vi "Flow vs Int Fac Input.vi"() -> ()   [LabVIEW 2009]
uses:
  Intellifaucet/Intellfaucet Mode.ctl
  ChannelSettings.ctl
  <vilib>/Analysis/NI_AALBase.lvlib
panel:
  out "Results(Flow,Percent)":dbl[][](array[numeric])
  out "Flowrate":dbl(graph)
  out "Percent Input":i32
  out "error out":errorcluster
  out "Flow":dbl
  in  "seconds to wait between reported averages":u32=15
  in  "error in (no error)":errorcluster
  in  "Semiphore":T1
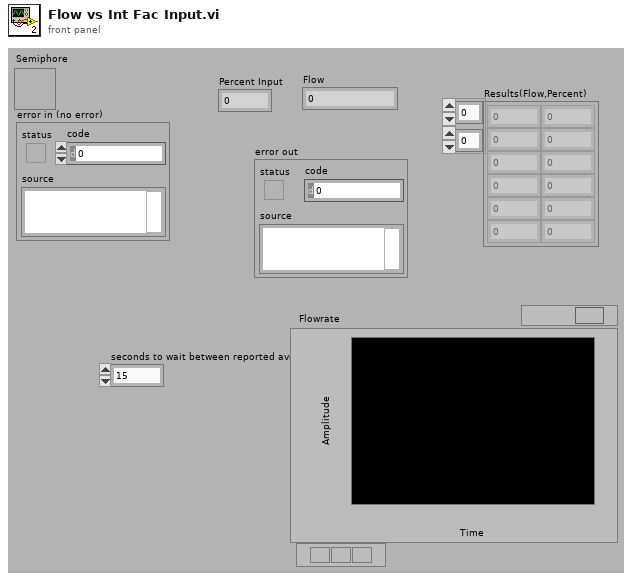
[diagram p1: front panel]
types:
  T1 = typedef "Semaphore RefNum" = refnum<k1>
  T2 = typedef "Intellfaucet Mode.ctl" = enum16{"Adjust Temp", "Adjust Flow", "Start Flow", "Stop Flow"}
  T3 = typedef "ChannelSettings.ctl" = u32
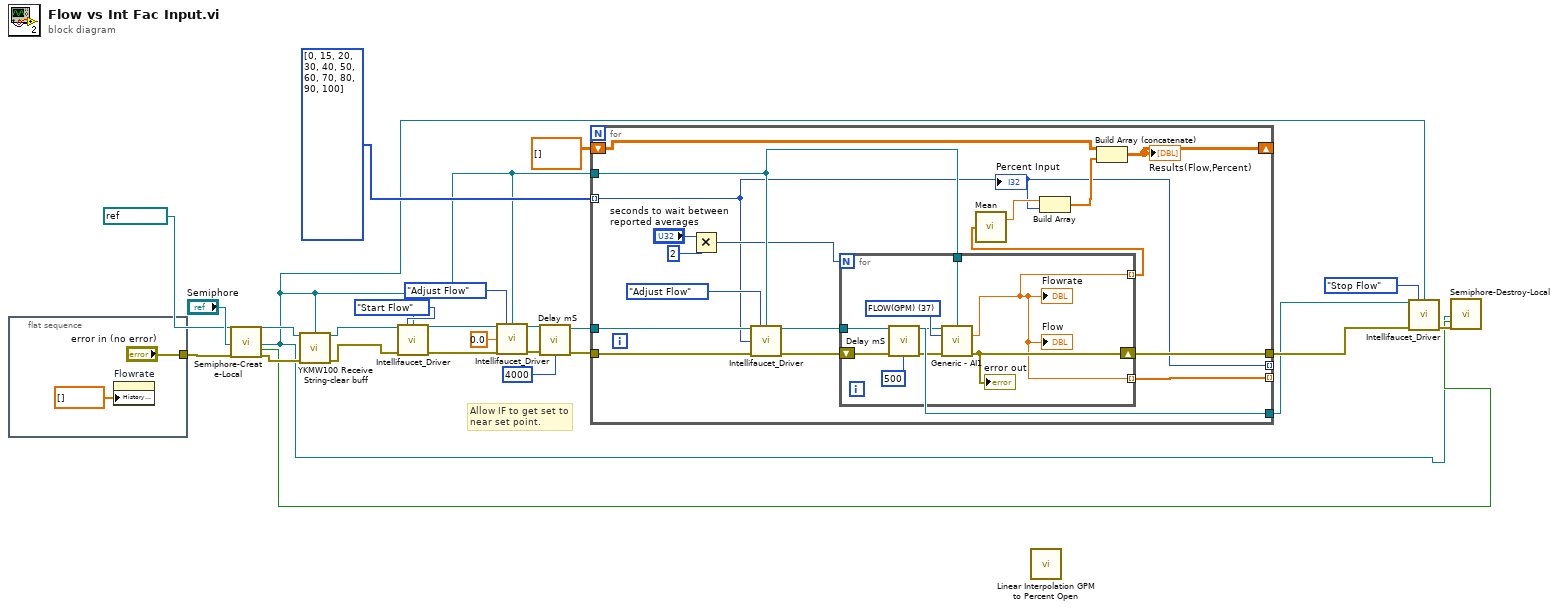
[diagram p0: block diagram]
diagram:
  # "Allow IF to get set to\nnear set point."
  n1 = flat-sequence {
    tunnel: ["error in (no error)"] -> w22
    frame #0 {
      n2 = property on="Flowrate" class="WFChart (strict)"("History Data"=dbl[] []) -> ()  [unwired: 2 in, 2 out]
    }
  }
  n3 = call "Semiphore-Create-Local.vi"("Semiphore"="Semiphore", "error in (no error)"=w22) -> ("semaphore"=w4:T1, "Local?"=w13:bool, "error out"=w15:errorcluster)  [unwired: 15 in]
  n4 = call "YKMW100 Receive String-clear buff.vi"("VISA session"=refnum<visa-resource-name> "MW100" ("MW100"), "Semiphore"=w4, "error in (no error)"=w15) -> ("dup VISA session"=w11:refnum<visa-resource-name>, "error out"=w14:errorcluster)  [unwired: 10 in, 1 out]
  n5 = call "Intellifaucet_Driver.vi"("VISA session"=w11, "Mode"=Intellfaucet_Mode."Start Flow", "Semiphore"=w4, "Error In"=w14) -> ("VISA session out"=w5:refnum<visa-resource-name>, "Error Out"=w10:errorcluster)  [unwired: 10 in]
  n6 = call "Intellifaucet_Driver.vi"("VISA session"=w5, "Mode"=Intellfaucet_Mode."Adjust Flow", "Semiphore"=w4, "Percent Flow"=0.0, "Error In"=w10) -> ("VISA session out"=w7:refnum<visa-resource-name>, "Error Out"=w9:errorcluster)  [unwired: 9 in]
  n7 = call "Delay mS.vi"("Error In"=w9, "milliseconds to wait"=u32 4000) -> ("Error Out"=w8:errorcluster)  [unwired: 13 in]
  n8 = for {
    tunnel: [w37] -> _ mode=indexing
    tunnel: w8 -> [w40]
    tunnel: w4 -> [w39]
    tunnel: [w28] -> _ mode=indexing
    tunnel: [w42] -> w18
    tunnel: i32[] [0, 15, 20, 30, 40, 50, 60, 70, 80, 90, 100] -> [w28] mode=indexing
    tunnel: [w36] -> w17
    tunnel: w7 -> [w35]
    shift-right: [w27] -> _
    shift-left: dbl[][] [] -> [w26]
    n9 = Multiply(x="seconds to wait between reported averages", y=u32 2) -> (x*y=w32:u32)
    n10 = call "Intellifaucet_Driver.vi"("VISA session"=w35, "Mode"=Intellfaucet_Mode."Adjust Flow", "Semiphore"=w39, "Percent Flow"=w28, "Error In"=w40) -> ("VISA session out"=w36:refnum<visa-resource-name>, "Error Out"=w41:errorcluster)  [unwired: 9 in]
    n11 = for {
      N: w32 -> [_]
      tunnel: w39 -> [w46]
      tunnel: [w43] -> w37 mode=indexing
      tunnel: w36 -> [w45]
      shift-right: [w48] -> w42
      shift-left: w41 -> [w47]
      tunnel: [w43] -> w31 mode=indexing
      w50 = T3 37 items=["4-20_OUT", "Pres_HI1", "Pres_HI2", "Pres_LOW", "Pres_PIN", "HEATER_TOP", "HEATER_BOT", "T_Shell", "FLOWMETER", "WATT_SENSE", "WH_TICK", "Tc_1", "Tc_2", "Tc_3", "Tc_4", "Tc_5", "Tc_6", "Tc_down", "T_Shell_2", "T_Shell_3", "T_Shell_4", "RTD_IN", "RTD_OUT", "RTD_AMB", "INTF_TEMPFLO", "INTF_READY", "INTF_START", "INTF_STOP", "DRM_LOW", "DRM_HIGH", "PWR_MAIN", "VLV_DUMP", "VLV_OUT", "VLV_IN", "WATT_HOURS", "FLOW(SAMPLE)", "GALLONS", "FLOW(GPM)"] ("Channel_Enum")
      n12 = call "Delay mS.vi"("Error In"=w47, "milliseconds to wait"=u32 500) -> ("Error Out"=w49:errorcluster)  [unwired: 13 in]
      n13 = call "Generic - AI1.vi"("MW100"=w45, "Semiphore"=w46, "Channel_Enum"=w50, "Error In"=w49) -> ("Value"=w43:dbl, "Error Out"=w48:errorcluster)  [unwired: 9 in, 1 out]
      "Flow" <- w43
      "error out" <- w48
      "Flowrate" <- w43
    }
    n14 = call <vilib>:"Mean.vi"("X"=w31) -> ("mean"=w29:dbl)  [unwired: 1 out]
    n15 = Build Array(w29, w28) -> (w30:dbl[])
    n16 = Build Array (concatenate)(w26, w30) -> (w27:dbl[][])
    "Results(Flow,Percent)" <- w27
    "Percent Input" <- w28
  }
  n17 = call "Linear Interpolation GPM to Percent Open.vi"() -> ()  [unwired: 11 in, 1 out]
  n18 = call "Intellifaucet_Driver.vi"("VISA session"=w17, "Mode"=Intellfaucet_Mode."Stop Flow", "Semiphore"=w4, "Error In"=w18) -> ("Error Out"=w20:errorcluster)  [unwired: 10 in, 1 out]
  n19 = call "Semiphore-Destroy-Local.vi"("Semiphore"=w4, "Local?"=w13, "error in (no error)"=w20) -> ()  [unwired: 16 in, 1 out]
